vi "LOERN_GenerateCode.vi"(0 "XRef":T11, 1 "Terms":T8, 2 "Diagram":T7, 3 "State In":T1={"Inputs"=1, "SelectedIndex"=1, "ClassInfo"=[]}) -> (14 "Generated Code?":T6, 15 "Reply":T4, 16 "Fatal Error Out":T3, 17 "State Out":T1={"Inputs"=1, "SelectedIndex"=1, "ClassInfo"=[]})   [LabVIEW 2016, in "LV Object Event Registration Node.xnode"]
uses:
  LV Object Event Registration Node.xnode
  <vilib>/XNodeSupport/XNodeXNodeRef.ctl
  <vilib>/XNodeSupport/XNodeTermIDPairs.ctl
  <vilib>/XNodeSupport/XNodeTermIDPair.ctl
  <vilib>/XNodeSupport/XNodeTermRef.ctl
  <vilib>/XNodeSupport/XNodeString.ctl
  <vilib>/XNodeSupport/XNodeTopLevelDiagramRef.ctl
  LOERN_State.ctl
  LOERN_ClassInfo.ctl
  <vilib>/XNodeSupport/XNodeBool.ctl
  <vilib>/XNodeSupport/XNodeStringArray.ctl
  <vilib>/XNodeSupport/XNodeErrorCluster.ctl
  <vilib>/XNodeSupport/NI_XNodeSupport.lvlib
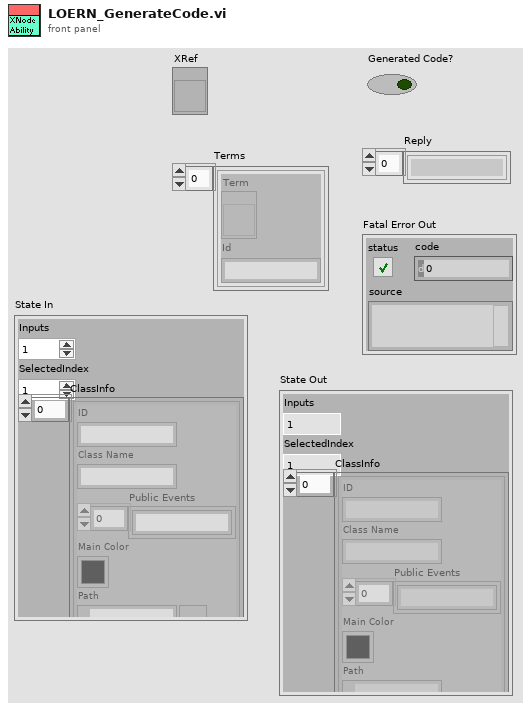
[diagram p1: front panel]
types:
  T1 = typedef "LV Object Event Registration Node.xnode/LOERN_State.ctl" = cluster{"Inputs":u16, "SelectedIndex":i16, "ClassInfo":T2[]}
  T2 = typedef "LV Object Event Registration Node.xnode/LOERN_ClassInfo.ctl" = cluster{"ID":string, "Class Name":string, "Public Events":string[], "Main Color":u32, "Path":path}
  T3 = typedef "NI_XNodeSupport.lvlib/XNodeErrorCluster.ctl" = errorcluster
  T4 = typedef "NI_XNodeSupport.lvlib/XNodeStringArray.ctl" = T5[]
  T5 = typedef "NI_XNodeSupport.lvlib/XNodeString.ctl" = string
  T6 = typedef "NI_XNodeSupport.lvlib/XNodeBool.ctl" = bool
  T7 = typedef "NI_XNodeSupport.lvlib/XNodeTopLevelDiagramRef.ctl" = refnum<vi>
  T8 = typedef "NI_XNodeSupport.lvlib/XNodeTermIDPairs.ctl" = T9[]
  T9 = typedef "NI_XNodeSupport.lvlib/XNodeTermIDPair.ctl" = cluster{"Term":T10, "Id":T5}
  T10 = typedef "NI_XNodeSupport.lvlib/XNodeTermRef.ctl" = refnum<vi>
  T11 = typedef "NI_XNodeSupport.lvlib/XNodeXNodeRef.ctl" = refnum<vi>
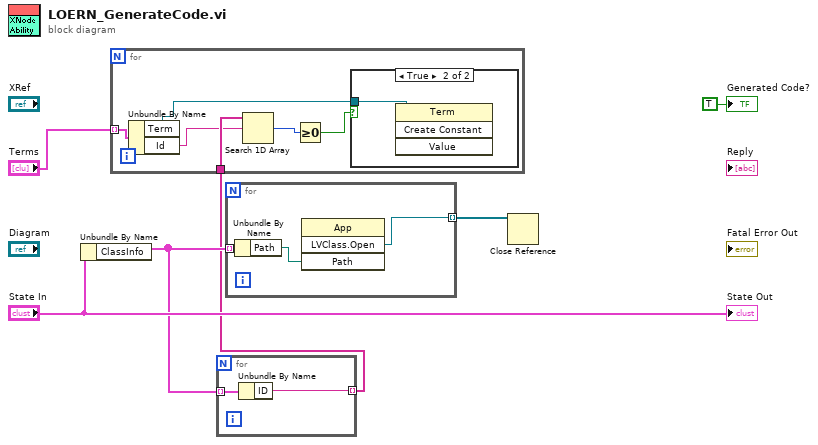
[diagram p0: block diagram]
diagram:
  n1 = Unbundle By Name("State In") -> ("ClassInfo"=w2:T2[])
  n2 = for {
    tunnel: w2 -> [w8] mode=indexing
    tunnel: [w7] -> w1 mode=indexing
    n3 = Unbundle By Name(w8) -> ("ID"=w7:string)
  }
  n4 = for {
    tunnel: "Terms" -> [w13] mode=indexing
    tunnel: w1 -> [w14]
    n5 = Unbundle By Name(w13) -> ("Term"=w10:T10, "Id"=w12:T5)
    n6 = Search 1D Array(1D array=w14, element=w12) -> (index of element=w11:i32)  [unwired: 1 in]
    n7 = Greater Or Equal To 0?(x=w11) -> (x >= 0?=w9:bool)
    n8 = case shown="True" w9 {
      tunnel: w10 -> [_ w15]
      frame False {
      }
      frame True {
        n9 = invoke class="Term" method="Create Constant"(reference=w15) -> ()  [unwired: 3 in, 4 out]
      }
    }
  }
  n10 = for {
    tunnel: w2 -> [w18] mode=indexing
    tunnel: [w16] -> w5 mode=indexing
    n11 = Unbundle By Name(w18) -> ("Path"=w17:path)
    n12 = invoke class="App" method="LVClass.Open"("Path"=w17) -> ("LVClass.Open"=w16:refnum<vi>)  [unwired: 3 in, 3 out]
  }
  n13 = Close Reference(reference=w5) -> ()  [unwired: 1 in, 1 out]
  "Generated Code?" <- T6 TRUE ("Generated Code?")
  "State Out" <- "State In"
